vi "CRYProject Editor PIC Change State.vi"(10 "bChangeState":bool) -> ()   [LabVIEW 2013]
uses:
  CRYProject Editor Global.vi
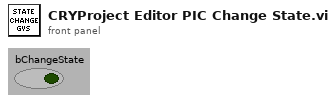
[diagram p1: front panel]
types:
  T1 = typedef "CRYTS.ctl" = cluster{"No.TS":u16, "TS File Path":path, "TS Name":string, "EditStepName":string, "Steps":T2[], "New State":bool, "Change State":bool, "Flattened CurveLib Data":string, "Document Data":string, "EditStepNo":u16, "Operator Start File":string, "Sequence Type":string, "Sequence Language":string}
  T2 = typedef "CRYStep.ctl" = cluster{"No.VI":i32, "Category":string, "StepName":string, "Seq setup flattened":string, "Comment":string, "Steps config.":bool[], "Jump config":i32[], "Start":dbl, "Increment":dbl, "Name":string, "Unit":string, "Y data":u16, "Y prefix":string, "Y dB ref":dbl, "Y unit":string, "Repeat State Array":cluster{"Start":dbl, "Increment":dbl, "Count":i32, "Num":i32}[]}
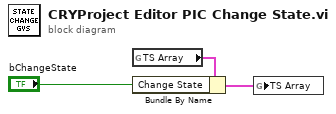
[diagram p0: block diagram]
diagram:
  n1 = global read "CRYProject Editor Global.vi" "TS Array"() -> (w3:T1)
  n2 = Bundle By Name(cluster=w3, "Change State"="bChangeState") -> (w2:T1)
  n3 = global write "CRYProject Editor Global.vi" "TS Array"(w2) -> ()
